vi "lijn volgen.vi"() -> (10 "staat op stopstreep":bool, 11 "lijn gedetecteerd":bool)   [LabVIEW 2019]
uses:
  <vilib>/myRIO/Common/Instrument Driver Framework/Utilities/typedefs/Analog Scaling Constants.ctl
  <vilib>/myRIO/Common/Instrument Driver Framework/Utilities/typedefs/Analog Scaling Constants List.ctl
  <vilib>/myRIO/Common/Instrument Driver Framework/myRIO v1.0/AO/typedefs/AO Channels Enum.ctl
  <vilib>/myRIO/Common/Instrument Driver Framework/myRIO v1.0/AO/typedefs/AO Channels List.ctl
  <vilib>/myRIO/Common/Instrument Driver Framework/Utilities/typedefs/Generic FPGA Reference.ctl
  <vilib>/myRIO/Common/Instrument Driver Framework/Utilities/typedefs/myRIO v1.0 Reference.ctl
  <vilib>/myRIO/Common/Instrument Driver Framework/Utilities/typedefs/Hardware Version Enum.ctl
  <vilib>/myRIO/Common/Instrument Driver Framework/Utilities/typedefs/myRIO Generic Hardware Reference.ctl
  <vilib>/myRIO/Instrument Drivers/Onboard IO/AO/typedefs/AO Reference.ctl
  <vilib>/myRIO/Instrument Drivers/Onboard IO/AO/AO.lvlib
  <vilib>/myRIO/Instrument Drivers/Onboard IO/AO/vis/Write.vi
  <vilib>/userDefined/High Color/nirio_resource_hc.ctl
  <vilib>/myRIO/Common/Instrument Driver Framework/myRIO v1.0/AO/vis/myRIO v1.1 Open AO.vi
  <vilib>/myRIO/Instrument Drivers/Onboard IO/AO/vis/myRIO AO Open.xnode
  <vilib>/myRIO/Common/Instrument Driver Framework/Utilities/vis/Is FPGA Ref Available.vi
  <vilib>/myRIO/Express VI/Onboard IO/AO/AO Express VI.xnode
  <vilib>/myRIO/Common/Instrument Driver Framework/myRIO v1.0/AI/typedefs/AI Channels Enum.ctl
  <vilib>/myRIO/Common/Instrument Driver Framework/myRIO v1.0/AI/typedefs/AI Channels List.ctl
  <vilib>/myRIO/Instrument Drivers/Onboard IO/AI/typedefs/AI Reference.ctl
  <vilib>/myRIO/Instrument Drivers/Onboard IO/AI/AI.lvlib
  <vilib>/myRIO/Instrument Drivers/Onboard IO/AI/vis/Read.vi
  <vilib>/myRIO/Common/Instrument Driver Framework/myRIO v1.0/AI/vis/myRIO v1.1 Open AI.vi
  <vilib>/myRIO/Instrument Drivers/Onboard IO/AI/vis/myRIO AI Open.xnode
  <vilib>/myRIO/Express VI/Onboard IO/AI/AI Express VI.xnode
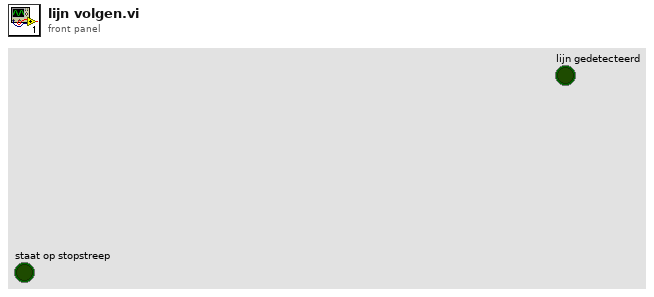
[diagram p1: front panel]
types:
  T1 = typedef "AO.lvlib/AO Reference.ctl" = cluster{"myRIO Reference":T2, "AO Channel List":T6, "AO Scaling Constant List":T8}
  T2 = typedef "myRIO Generic Hardware Reference.ctl" = cluster{"myRIO Model":T3, "myRIO Hardware Reference":T4}
  T3 = typedef "Hardware Version Enum.ctl" = enum16{"Unknown", "myRIO-1900", "myRIO-1950", "roboRIO", "NI ELVIS RIO CM", "ELVIS III"}
  T4 = typedef "myRIO v1.0 Reference.ctl" = cluster{"Generic FPGA Reference":T5, "Allow multiple opens":bool}
  T5 = typedef "Generic FPGA Reference.ctl" = refnum<k20>
  T6 = typedef "AO Channels List.ctl" = T7[]
  T7 = typedef "AO Channels Enum.ctl" = enum16{"Not Connected", "AudioOut/Left", "AudioOut/Right", "C/AO0", "C/AO1", "A/AO0", "A/AO1", "B/AO0", "B/AO1"}
  T8 = typedef "Analog Scaling Constants List.ctl" = T9[]
  T9 = typedef "Analog Scaling Constants.ctl" = cluster{"LSB Weight (Volts)":dbl, "Offset (Volts)":dbl, "Signed?":bool}
  T10 = typedef "nirio_resource_hc.ctl" = tag
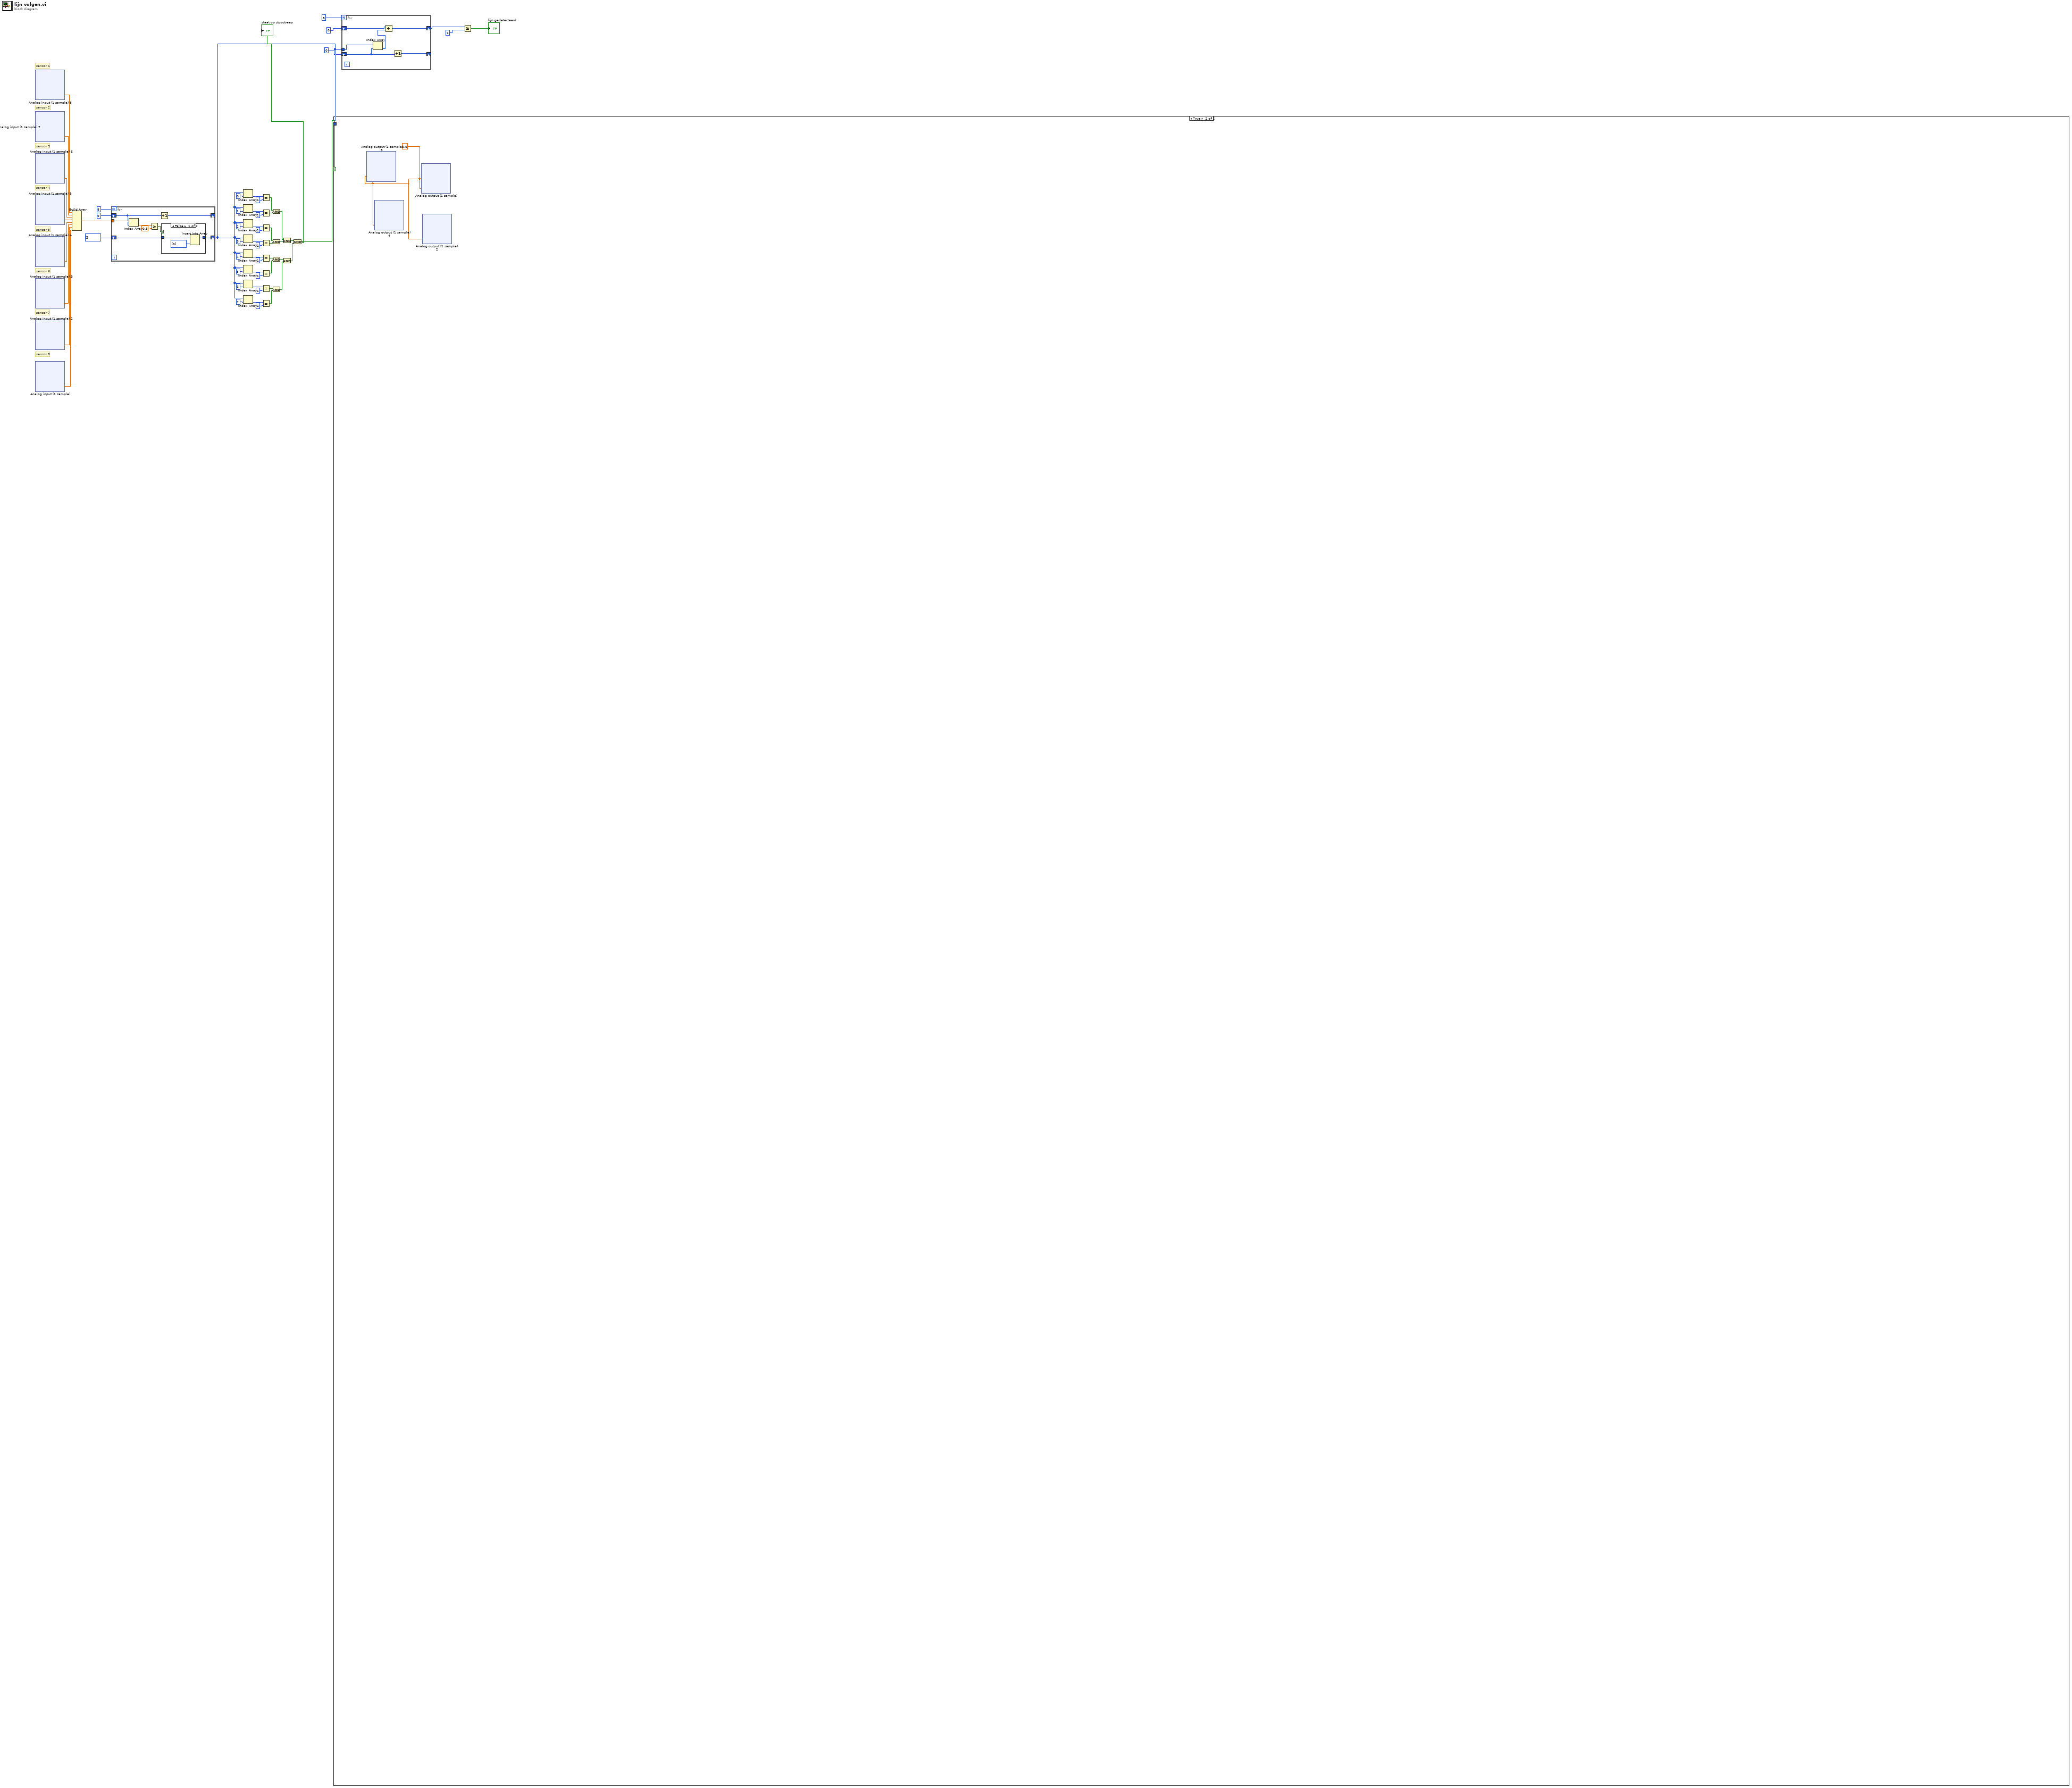
[diagram p0: block diagram]
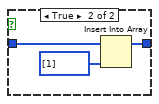
[diagram p2: hidden frame]
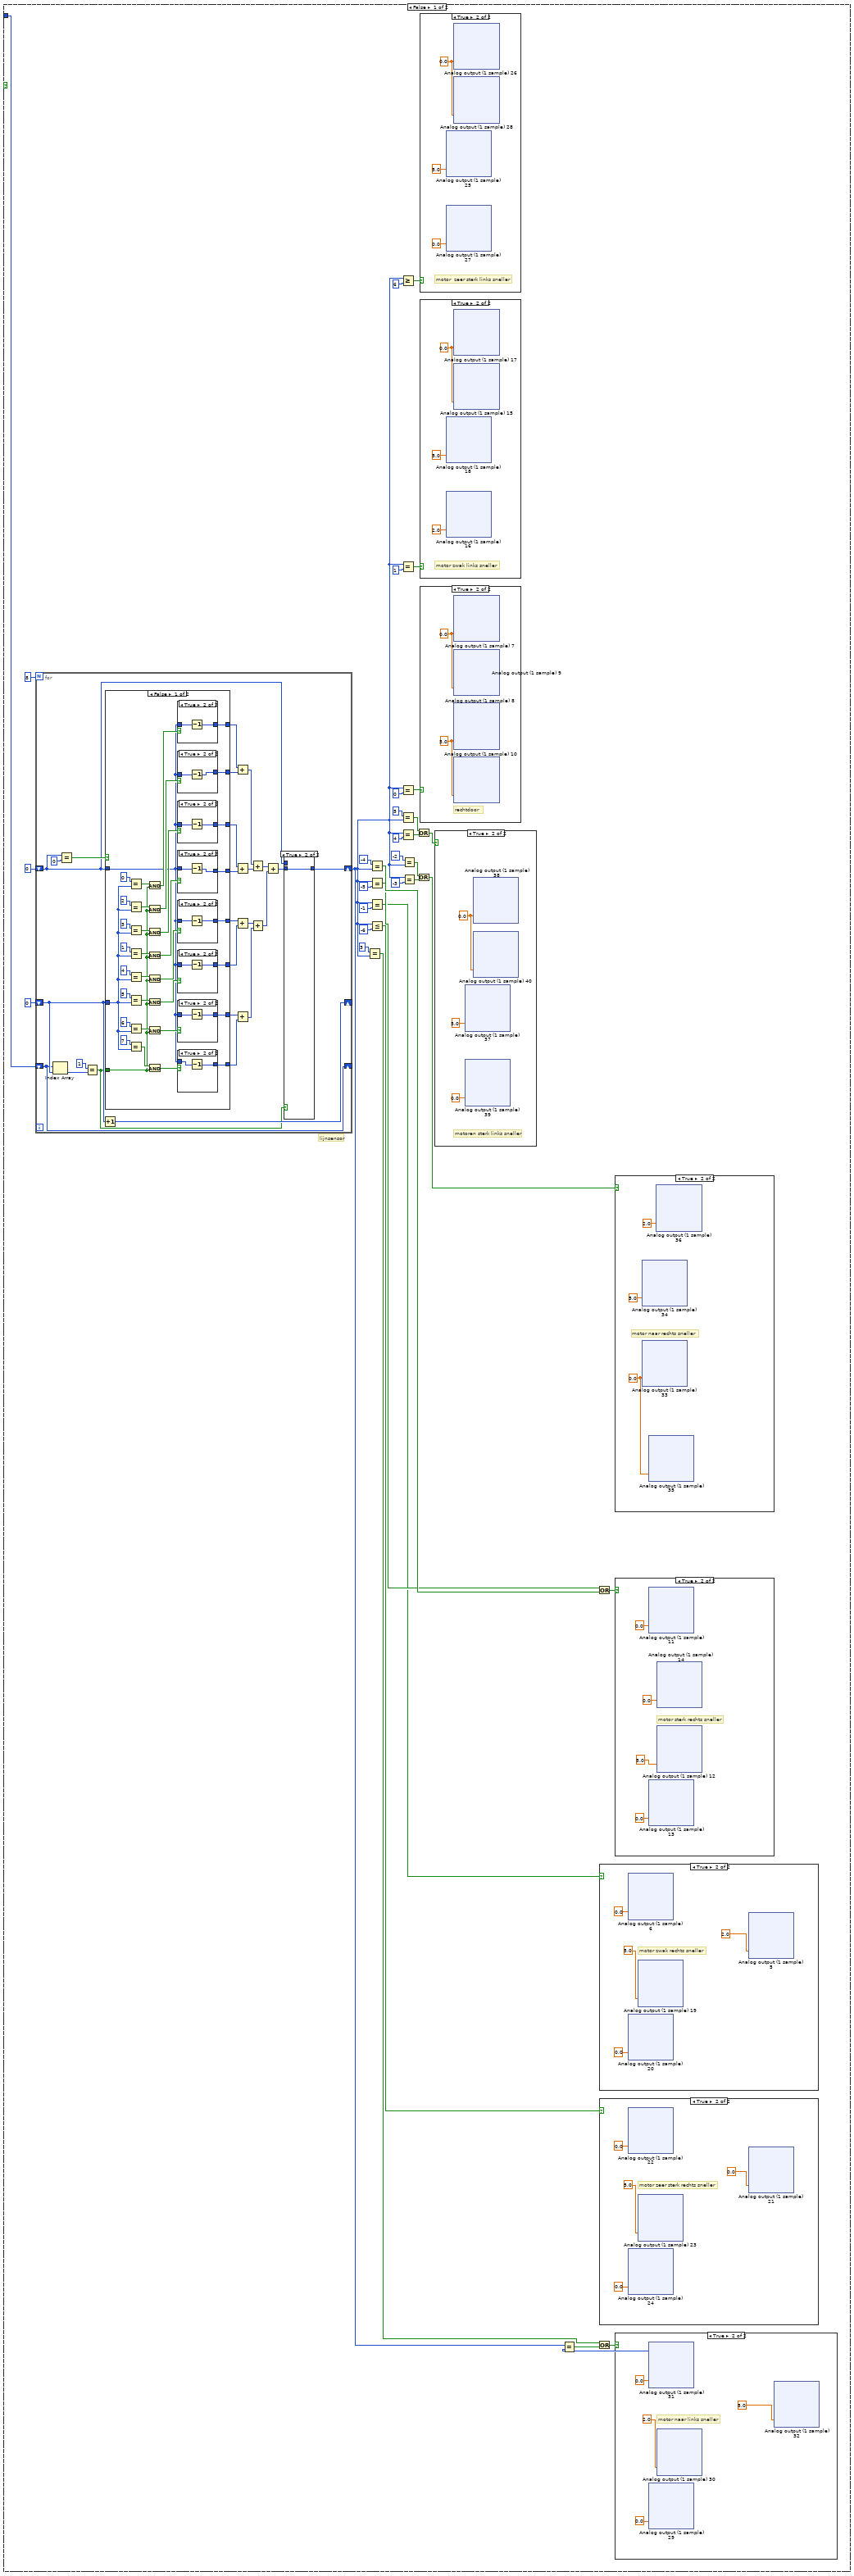
[diagram p3: hidden frame]
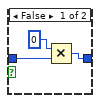
[diagram p14: hidden frame]
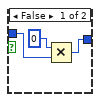
[diagram p15: hidden frame]
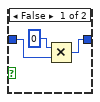
[diagram p16: hidden frame]
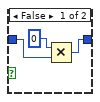
[diagram p17: hidden frame]
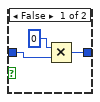
[diagram p18: hidden frame]
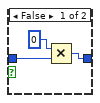
[diagram p19: hidden frame]
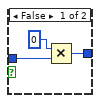
[diagram p20: hidden frame]
diagram:
  # "sensor 8"
  # "sensor 7"
  # "sensor 6"
  # "sensor 5"
  # "sensor 4"
  # "sensor 3"
  # "sensor 2"
  # "sensor 1"
  n1 = xnode "Analog input (1 sample) 8"() -> ("A/AI3 (Pin 9)"=w16:dbl)  [unwired: 1 in, 1 out]
  n2 = xnode "Analog input (1 sample) 7"() -> ("A/AI2 (Pin 7)"=w15:dbl)  [unwired: 1 in, 1 out]
  n3 = xnode "Analog input (1 sample) 6"() -> ("A/AI1 (Pin 5)"=w14:dbl)  [unwired: 1 in, 1 out]
  n4 = xnode "Analog input (1 sample) 5"() -> ("A/AI0 (Pin 3)"=w13:dbl)  [unwired: 1 in, 1 out]
  n5 = xnode "Analog input (1 sample) 4"() -> ("B/AI3 (Pin 9)"=w12:dbl)  [unwired: 1 in, 1 out]
  n6 = xnode "Analog input (1 sample) 3"() -> ("B/AI2 (Pin 7)"=w11:dbl)  [unwired: 1 in, 1 out]
  n7 = xnode "Analog input (1 sample) 2"() -> ("A/AI1 (Pin 5)"=w10:dbl)  [unwired: 1 in, 1 out]
  n8 = xnode "Analog input (1 sample)"() -> ("B/AI0 (Pin 3)"=w9:dbl)  [unwired: 1 in, 1 out]
  n9 = Build Array(w16, w15, w14, w13, w12, w11, w10, w9) -> (w8:dbl[])
  n10 = for {
    N: 8 -> [_]
    shift-right: [w65] -> w7
    shift-left: i32[] [] -> [w66]
    shift-right: [w64] -> _
    shift-left: 0 -> [w62]
    tunnel: w8 -> [w63]
    n11 = Index Array(array=w63, index=w62) -> (element=w60:dbl)
    n12 = Greater Or Equal?(x=w60, y=0.3) -> (x >= y?=w61:bool)
    n13 = Increment(x=w62) -> (x+1=w64:i32)
    n14 = case shown="False" w61 {
      tunnel: w66 -> [w68 w70]
      tunnel: [w69 w72] -> w65
      frame False {
        n15 = Insert Into Array(array=w68, new element=i32[] [0]) -> (w69:i32[])  [unwired: 1 in]
      }
      frame True {
        n16 = Insert Into Array(array=w70, new element=i32[] [1]) -> (w72:i32[])  [unwired: 1 in]
      }
    }
  }
  n17 = Index Array(array=w7, index=0) -> (element=w38:i32)
  n18 = Index Array(array=w7, index=1) -> (element=w17:i32)
  n19 = Index Array(array=w7, index=2) -> (element=w23:i32)
  n20 = Index Array(array=w7, index=3) -> (element=w20:i32)
  n21 = Index Array(array=w7, index=4) -> (element=w26:i32)
  n22 = Index Array(array=w7, index=5) -> (element=w29:i32)
  n23 = Index Array(array=w7, index=6) -> (element=w32:i32)
  n24 = Index Array(array=w7, index=7) -> (element=w35:i32)
  n25 = Equal?(x=w38, y=1) -> (x = y?=w41:bool)
  n26 = Equal?(x=w17, y=1) -> (x = y?=w42:bool)
  n27 = Equal?(x=w23, y=1) -> (x = y?=w43:bool)
  n28 = Equal?(x=w20, y=1) -> (x = y?=w44:bool)
  n29 = Equal?(x=w26, y=1) -> (x = y?=w45:bool)
  n30 = Equal?(x=w29, y=1) -> (x = y?=w46:bool)
  n31 = Equal?(x=w32, y=1) -> (x = y?=w47:bool)
  n32 = Equal?(x=w35, y=1) -> (x = y?=w48:bool)
  n33 = And(x=w41, y=w42) -> (x .and. y?=w49:bool)
  n34 = And(x=w43, y=w44) -> (x .and. y?=w50:bool)
  n35 = And(x=w45, y=w46) -> (x .and. y?=w51:bool)
  n36 = And(x=w47, y=w48) -> (x .and. y?=w52:bool)
  n37 = And(x=w49, y=w50) -> (x .and. y?=w53:bool)
  n38 = And(x=w51, y=w52) -> (x .and. y?=w54:bool)
  n39 = And(x=w53, y=w54) -> (x .and. y?=w58:bool)
  "staat op stopstreep" <- w58
  n40 = case shown="True" w58 {
    tunnel: w7 -> [w76 _]
    frame False {
      # "lijnsensor"
      n41 = for {
        N: 8 -> [_]
        shift-right: [w1480] -> _
        shift-left: 0 -> [w1494]
        shift-right: [w1472] -> w73
        shift-left: 0 -> [w1473]
        shift-right: [w1485] -> _
        shift-left: w76 -> [w1485]
        n42 = Index Array(array=w1485, index=w1494) -> (element=w1484:i32)
        n43 = Equal?(x=w1473, y=0) -> (x = y?=w1481:bool)
        n44 = Equal?(x=1, y=w1484) -> (x = y?=w1471:bool)
        n45 = Increment(x=w1494) -> (x+1=w1480:i32)
        n46 = case shown="False" w1481 {
          tunnel: w1494 -> [w1504 w1590]
          tunnel: [w1498 w1589] -> w1493
          tunnel: [w1505 w1588] -> w1492
          tunnel: [w1506 w1587] -> w1491
          tunnel: [w1507 w1586] -> w1490
          tunnel: w1473 -> [w1497 w1585]
          tunnel: w1471 -> [w1503 w1576]
          tunnel: [w1501 w1575] -> w1479
          tunnel: [w1502 w1574] -> w1478
          tunnel: [w1499 w1573] -> w1476
          tunnel: [w1500 w1572] -> w1475
          frame False {
            n47 = Equal?(x=0, y=w1504) -> (x = y?=w1524:bool)
            n48 = Equal?(x=2, y=w1504) -> (x = y?=w1530:bool)
            n49 = Equal?(x=3, y=w1504) -> (x = y?=w1531:bool)
            n50 = Equal?(x=1, y=w1504) -> (x = y?=w1516:bool)
            n51 = Equal?(x=4, y=w1504) -> (x = y?=w1528:bool)
            n52 = Equal?(x=5, y=w1504) -> (x = y?=w1529:bool)
            n53 = Equal?(x=6, y=w1504) -> (x = y?=w1527:bool)
            n54 = Equal?(x=7, y=w1504) -> (x = y?=w1526:bool)
            n55 = And(x=w1524, y=w1503) -> (x .and. y?=w1508:bool)
            n56 = And(x=w1530, y=w1503) -> (x .and. y?=w1510:bool)
            n57 = And(x=w1531, y=w1503) -> (x .and. y?=w1511:bool)
            n58 = And(x=w1516, y=w1503) -> (x .and. y?=w1509:bool)
            n59 = And(x=w1528, y=w1503) -> (x .and. y?=w1512:bool)
            n60 = And(x=w1529, y=w1503) -> (x .and. y?=w1513:bool)
            n61 = And(x=w1527, y=w1503) -> (x .and. y?=w1514:bool)
            n62 = And(x=w1526, y=w1503) -> (x .and. y?=w1515:bool)
            n63 = case shown="True" w1508 {
              tunnel: [w1533 w1536] -> w1502
              tunnel: w1497 -> [w1532 w1535]
              frame False {
                n64 = Multiply(x=0, y=w1532) -> (x*y=w1533:i32)
              }
              frame True {
                n65 = Decrement(x=w1535) -> (x-1=w1536:i32)
              }
            }
            n66 = case shown="True" w1510 {
              tunnel: [w1564 w1565] -> w1501
              tunnel: w1497 -> [w1563 w1566]
              frame False {
                n67 = Multiply(x=0, y=w1563) -> (x*y=w1564:i32)
              }
              frame True {
                n68 = Decrement(x=w1566) -> (x-1=w1565:i32)
              }
            }
            n69 = case shown="True" w1511 {
              tunnel: [w1558 w1561] -> w1500
              tunnel: w1497 -> [w1557 w1560]
              frame False {
                n70 = Multiply(x=0, y=w1557) -> (x*y=w1558:i32)
              }
              frame True {
                n71 = Decrement(x=w1560) -> (x-1=w1561:i32)
              }
            }
            n72 = case shown="True" w1509 {
              tunnel: [w1568 w1571] -> w1499
              tunnel: w1497 -> [w1567 w1570]
              frame False {
                n73 = Multiply(x=0, y=w1567) -> (x*y=w1568:i32)
              }
              frame True {
                n74 = Decrement(x=w1570) -> (x-1=w1571:i32)
              }
            }
            n75 = case shown="True" w1512 {
              tunnel: [w1553 w1556] -> w1498
              tunnel: w1497 -> [w1552 w1555]
              frame False {
                n76 = Multiply(x=0, y=w1552) -> (x*y=w1553:i32)
              }
              frame True {
                n77 = Decrement(x=w1555) -> (x-1=w1556:i32)
              }
            }
            n78 = case shown="True" w1513 {
              tunnel: [w1543 w1546] -> w1505
              tunnel: w1497 -> [w1542 w1545]
              frame False {
                n79 = Multiply(x=0, y=w1542) -> (x*y=w1543:i32)
              }
              frame True {
                n80 = Decrement(x=w1545) -> (x-1=w1546:i32)
              }
            }
            n81 = case shown="True" w1514 {
              tunnel: [w1548 w1551] -> w1506
              tunnel: w1497 -> [w1547 w1550]
              frame False {
                n82 = Multiply(x=0, y=w1547) -> (x*y=w1548:i32)
              }
              frame True {
                n83 = Decrement(x=w1550) -> (x-1=w1551:i32)
              }
            }
            n84 = case shown="True" w1515 {
              tunnel: [w1537 w1541] -> w1507
              tunnel: w1497 -> [w1538 w1540]
              frame False {
                n85 = Multiply(x=0, y=w1538) -> (x*y=w1537:i32)
              }
              frame True {
                n86 = Decrement(x=w1540) -> (x-1=w1541:i32)
              }
            }
          }
          frame True {
            n87 = Equal?(x=0, y=w1590) -> (x = y?=w1599:bool)
            n88 = Equal?(x=1, y=w1590) -> (x = y?=w1591:bool)
            n89 = Equal?(x=2, y=w1590) -> (x = y?=w1605:bool)
            n90 = Equal?(x=3, y=w1590) -> (x = y?=w1606:bool)
            n91 = Equal?(x=4, y=w1590) -> (x = y?=w1603:bool)
            n92 = Equal?(x=5, y=w1590) -> (x = y?=w1604:bool)
            n93 = Equal?(x=6, y=w1590) -> (x = y?=w1602:bool)
            n94 = Equal?(x=7, y=w1590) -> (x = y?=w1601:bool)
            n95 = And(x=w1599, y=w1576) -> (x .and. y?=w1577:bool)
            n96 = And(x=w1591, y=w1576) -> (x .and. y?=w1578:bool)
            n97 = And(x=w1605, y=w1576) -> (x .and. y?=w1579:bool)
            n98 = And(x=w1606, y=w1576) -> (x .and. y?=w1580:bool)
            n99 = And(x=w1603, y=w1576) -> (x .and. y?=w1581:bool)
            n100 = And(x=w1604, y=w1576) -> (x .and. y?=w1582:bool)
            n101 = And(x=w1602, y=w1576) -> (x .and. y?=w1583:bool)
            n102 = And(x=w1601, y=w1576) -> (x .and. y?=w1584:bool)
            n103 = case shown="True" w1577 {
              tunnel: w1585 -> [w1607 w1611]
              tunnel: [w1608 w1610] -> w1574
              frame False {
                n104 = Multiply(x=0, y=w1607) -> (x*y=w1608:i32)
              }
              frame True {
                n105 = Add(x=7, y=w1611) -> (x+y=w1610:i32)
              }
            }
            n106 = case shown="True" w1578 {
              tunnel: w1585 -> [w1647 w1650]
              tunnel: [w1648 w1651] -> w1575
              frame False {
                n107 = Multiply(x=0, y=w1647) -> (x*y=w1648:i32)
              }
              frame True {
                n108 = Add(x=5, y=w1650) -> (x+y=w1651:i32)
              }
            }
            n109 = case shown="True" w1579 {
              tunnel: w1585 -> [w1641 w1645]
              tunnel: [w1642 w1644] -> w1572
              frame False {
                n110 = Multiply(x=0, y=w1641) -> (x*y=w1642:i32)
              }
              frame True {
                n111 = Add(x=3, y=w1645) -> (x+y=w1644:i32)
              }
            }
            n112 = case shown="True" w1580 {
              tunnel: w1585 -> [w1637 w1640]
              tunnel: [w1636 w1639] -> w1573
              frame False {
                n113 = Multiply(x=0, y=w1637) -> (x*y=w1636:i32)
              }
              frame True {
                n114 = Increment(x=w1640) -> (x+1=w1639:i32)
              }
            }
            n115 = case shown="True" w1581 {
              tunnel: w1585 -> [w1631 w1635]
              tunnel: [w1632 w1634] -> w1589
              frame False {
                n116 = Multiply(x=0, y=w1631) -> (x*y=w1632:i32)
              }
              frame True {
                n117 = Decrement(x=w1635) -> (x-1=w1634:i32)
              }
            }
            n118 = case shown="True" w1582 {
              tunnel: w1585 -> [w1620 w1622]
              tunnel: [w1619 w1624] -> w1588
              frame False {
                n119 = Multiply(x=0, y=w1620) -> (x*y=w1619:i32)
              }
              frame True {
                n120 = Subtract(x=w1622, y=3) -> (x-y=w1624:i32)
              }
            }
            n121 = case shown="True" w1583 {
              tunnel: w1585 -> [w1626 w1628]
              tunnel: [w1625 w1629] -> w1587
              frame False {
                n122 = Multiply(x=0, y=w1626) -> (x*y=w1625:i32)
              }
              frame True {
                n123 = Subtract(x=w1628, y=5) -> (x-y=w1629:i32)
              }
            }
            n124 = case shown="True" w1584 {
              tunnel: w1585 -> [w1613 w1616]
              tunnel: [w1614 w1617] -> w1586
              frame False {
                n125 = Multiply(x=0, y=w1613) -> (x*y=w1614:i32)
              }
              frame True {
                n126 = Subtract(x=w1616, y=7) -> (x-y=w1617:i32)
              }
            }
          }
        }
        n127 = Add(x=w1478, y=w1479) -> (x+y=w1477:i32)
        n128 = Add(x=w1475, y=w1476) -> (x+y=w1474:i32)
        n129 = Add(x=w1493, y=w1492) -> (x+y=w1488:i32)
        n130 = Add(x=w1491, y=w1490) -> (x+y=w1489:i32)
        n131 = Add(x=w1477, y=w1474) -> (x+y=w1487:i32)
        n132 = Add(x=w1488, y=w1489) -> (x+y=w1486:i32)
        n133 = Add(x=w1487, y=w1486) -> (x+y=w1470:i32)
        n134 = case shown="True" w1471 {
          tunnel: w1473 -> [w1495 _]
          tunnel: [w1495 w1496] -> w1472
          tunnel: w1470 -> [_ w1496]
          frame False {
          }
          frame True {
          }
        }
      }
      n135 = Equal?(x=3, y=w73) -> (x = y?=w93:bool)
      n136 = Equal?(x=-4, y=w73) -> (x = y?=w83:bool)
      n137 = Equal?(x=w73, y=-5) -> (x = y?=w84:bool)
      n138 = Equal?(x=w73, y=-1) -> (x = y?=w81:bool)
      n139 = Less Or Equal?(x=w73, y=-6) -> (x <= y?=w79:bool)
      n140 = Greater Or Equal?(x=w73, y=6) -> (x >= y?=w102:bool)
      n141 = Equal?(x=w73, y=1) -> (x = y?=w103:bool)
      n142 = Equal?(x=w73, y=0) -> (x = y?=w74:bool)
      n143 = Equal?(x=5, y=w73) -> (x = y?=w97:bool)
      n144 = Equal?(x=w73, y=4) -> (x = y?=w98:bool)
      n145 = Equal?(x=-2, y=w73) -> (x = y?=w87:bool)
      n146 = Equal?(x=w73, y=-3) -> (x = y?=w88:bool)
      n147 = Or(x=w97, y=w98) -> (x .or. y?=w99:bool)
      n148 = Or(x=w87, y=w88) -> (x .or. y?=w80:bool)
      n149 = case shown="True" w102 {
        frame False {
        }
        frame True {
          w1319 = 0.0
          # "motor  zeer sterk links sneller"
          n150 = xnode "Analog output (1 sample) 25"("A/AO0 (Pin 2)"=5.0) -> ()  [unwired: 1 in, 1 out]
          n151 = xnode "Analog output (1 sample) 27"("B/AO0 (Pin 2)"=0.0) -> ()  [unwired: 1 in, 1 out]
          n152 = xnode "Analog output (1 sample) 26"("A/AO1 (Pin 4)"=w1319) -> ()  [unwired: 1 in, 1 out]
          n153 = xnode "Analog output (1 sample) 28"("B/AO1 (Pin 4)"=w1319) -> ()  [unwired: 1 in, 1 out]
        }
      }
      n154 = case shown="True" w103 {
        frame False {
        }
        frame True {
          w410 = 0.0
          # "motor zwak links sneller"
          n155 = xnode "Analog output (1 sample) 18"("A/AO0 (Pin 2)"=5.0) -> ()  [unwired: 1 in, 1 out]
          n156 = xnode "Analog output (1 sample) 16"("B/AO0 (Pin 2)"=2.0) -> ()  [unwired: 1 in, 1 out]
          n157 = xnode "Analog output (1 sample) 17"("A/AO1 (Pin 4)"=w410) -> ()  [unwired: 1 in, 1 out]
          n158 = xnode "Analog output (1 sample) 15"("B/AO1 (Pin 4)"=w410) -> ()  [unwired: 1 in, 1 out]
        }
      }
      n159 = case shown="True" w74 {
        frame False {
        }
        frame True {
          w109 = 0.0
          w108 = 5.0
          # "rechtdoor"
          n160 = xnode "Analog output (1 sample) 7"("B/AO1 (Pin 4)"=w109) -> ()  [unwired: 1 in, 1 out]
          n161 = xnode "Analog output (1 sample) 9"("A/AO1 (Pin 4)"=w109) -> ()  [unwired: 1 in, 1 out]
          n162 = xnode "Analog output (1 sample) 8"("B/AO0 (Pin 2)"=w108) -> ()  [unwired: 1 in, 1 out]
          n163 = xnode "Analog output (1 sample) 10"("A/AO0 (Pin 2)"=w108) -> ()  [unwired: 1 in, 1 out]
        }
      }
      n164 = case shown="True" w99 {
        frame False {
        }
        frame True {
          w1168 = 0.0
          # "motoren sterk links sneller"
          n165 = xnode "Analog output (1 sample) 37"("A/AO0 (Pin 2)"=5.0) -> ()  [unwired: 1 in, 1 out]
          n166 = xnode "Analog output (1 sample) 39"("B/AO0 (Pin 2)"=0.0) -> ()  [unwired: 1 in, 1 out]
          n167 = xnode "Analog output (1 sample) 38"("A/AO1 (Pin 4)"=w1168) -> ()  [unwired: 1 in, 1 out]
          n168 = xnode "Analog output (1 sample) 40"("B/AO1 (Pin 4)"=w1168) -> ()  [unwired: 1 in, 1 out]
        }
      }
      n169 = Equal?(x=w73, y=2) -> (x = y?=w94:bool)
      n170 = Or(x=w83, y=w84) -> (x .or. y?=w77:bool)
      n171 = Or(x=w93, y=w94) -> (x .or. y?=w91:bool)
      n172 = case shown="True" w81 {
        frame False {
        }
        frame True {
          # "motor zwak rechts sneller"
          n173 = xnode "Analog output (1 sample) 6"("A/AO1 (Pin 4)"=0.0) -> ()  [unwired: 1 in, 1 out]
          n174 = xnode "Analog output (1 sample) 20"("B/AO1 (Pin 4)"=0.0) -> ()  [unwired: 1 in, 1 out]
          n175 = xnode "Analog output (1 sample) 19"("B/AO0 (Pin 2)"=5.0) -> ()  [unwired: 1 in, 1 out]
          n176 = xnode "Analog output (1 sample) 5"("A/AO0 (Pin 2)"=2.0) -> ()  [unwired: 1 in, 1 out]
        }
      }
      n177 = case shown="True" w79 {
        frame False {
        }
        frame True {
          # "motor zeer sterk rechts sneller"
          n178 = xnode "Analog output (1 sample) 22"("A/AO1 (Pin 4)"=0.0) -> ()  [unwired: 1 in, 1 out]
          n179 = xnode "Analog output (1 sample) 24"("B/AO1 (Pin 4)"=0.0) -> ()  [unwired: 1 in, 1 out]
          n180 = xnode "Analog output (1 sample) 23"("B/AO0 (Pin 2)"=5.0) -> ()  [unwired: 1 in, 1 out]
          n181 = xnode "Analog output (1 sample) 21"("A/AO0 (Pin 2)"=0.0) -> ()  [unwired: 1 in, 1 out]
        }
      }
      n182 = case shown="True" w80 {
        frame False {
        }
        frame True {
          w866 = 0.0
          # "motor naar rechts sneller"
          n183 = xnode "Analog output (1 sample) 34"("B/AO0 (Pin 2)"=5.0) -> ()  [unwired: 1 in, 1 out]
          n184 = xnode "Analog output (1 sample) 33"("B/AO1 (Pin 4)"=w866) -> ()  [unwired: 1 in, 1 out]
          n185 = xnode "Analog output (1 sample) 35"("A/AO1 (Pin 4)"=w866) -> ()  [unwired: 1 in, 1 out]
          n186 = xnode "Analog output (1 sample) 36"("A/AO0 (Pin 2)"=2.0) -> ()  [unwired: 1 in, 1 out]
        }
      }
      n187 = case shown="True" w77 {
        frame False {
        }
        frame True {
          # "motor sterk rechts sneller"
          n188 = xnode "Analog output (1 sample) 11"("B/AO1 (Pin 4)"=0.0) -> ()  [unwired: 1 in, 1 out]
          n189 = xnode "Analog output (1 sample) 13"("A/AO1 (Pin 4)"=0.0) -> ()  [unwired: 1 in, 1 out]
          n190 = xnode "Analog output (1 sample) 14"("A/AO0 (Pin 2)"=0.0) -> ()  [unwired: 1 in, 1 out]
          n191 = xnode "Analog output (1 sample) 12"("B/AO0 (Pin 2)"=5.0) -> ()  [unwired: 1 in, 1 out]
        }
      }
      n192 = case shown="True" w91 {
        frame False {
        }
        frame True {
          # "motor naar links sneller"
          n193 = xnode "Analog output (1 sample) 31"("A/AO1 (Pin 4)"=0.0) -> ()  [unwired: 1 in, 1 out]
          n194 = xnode "Analog output (1 sample) 29"("B/AO1 (Pin 4)"=0.0) -> ()  [unwired: 1 in, 1 out]
          n195 = xnode "Analog output (1 sample) 30"("B/AO0 (Pin 2)"=2.0) -> ()  [unwired: 1 in, 1 out]
          n196 = xnode "Analog output (1 sample) 32"("A/AO0 (Pin 2)"=5.0) -> ()  [unwired: 1 in, 1 out]
        }
      }
    }
    frame True {
      w1653 = 0.0
      n197 = xnode "Analog output (1 sample) 3"("A/AO1 (Pin 4)"=w1653) -> ()  [unwired: 1 in, 1 out]
      n198 = xnode "Analog output (1 sample) 4"("B/AO1 (Pin 4)"=w1653) -> ()  [unwired: 1 in, 1 out]
      n199 = xnode "Analog output (1 sample)"("A/AO0 (Pin 2)"=w1653) -> ()  [unwired: 1 in, 1 out]
      n200 = xnode "Analog output (1 sample) 2"("B/AO0 (Pin 2)"=w1653) -> ()  [unwired: 1 in, 1 out]
    }
  }
  n201 = for {
    N: 8 -> [_]
    tunnel: w7 -> [w1807]
    shift-right: [w1806] -> _
    shift-left: 0 -> [w1805]
    shift-right: [w1802] -> w3
    shift-left: 0 -> [w1804]
    n202 = Index Array(array=w1807, index=w1805) -> (element=w1803:i32)
    n203 = Add(x=w1804, y=w1803) -> (x+y=w1802:i32)
    n204 = Increment(x=w1805) -> (x+1=w1806:i32)
  }
  n205 = Greater Or Equal?(x=w3, y=1) -> (x >= y?=→"lijn gedetecteerd":bool)
